vi "FGV Config.vi"(7 "Enum":enum16{"Read Config", "Save Config"}(ring)=enum."Save Config", 8 "error in":errorcluster, 10 "Config in":T1, 11 "config FName":string) -> (0 "error out":errorcluster, 2 "Config out":T1)   [LabVIEW 2012]
uses:
  controls/TP_Config.ctl
  <vilib>/Utility/config.llb/NI_LVConfig.lvlib
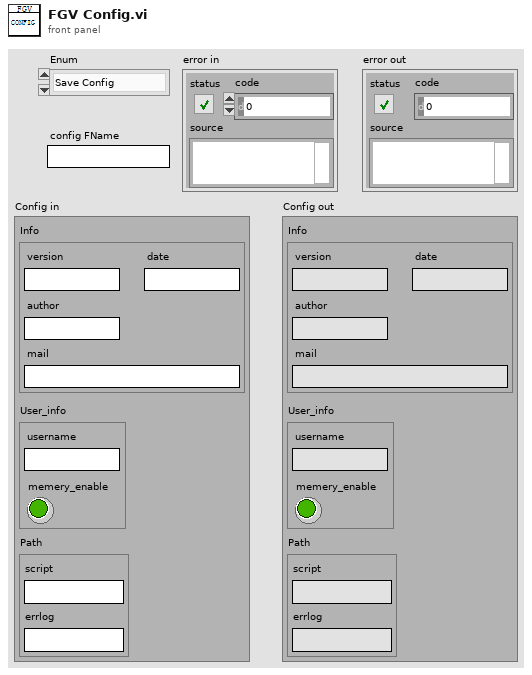
[diagram p1: front panel]
types:
  T1 = typedef "TP_Config.ctl" = cluster{"Info":cluster{"version":string, "date":string, "author":string, "mail":string}, "User_info":cluster{"username":string, "memery_enable":bool}, "Path":cluster{"script":string, "errlog":string}}
  T2 = typedef "NI_LVConfig.lvlib/Config Data RefNum.ctl" = refnum<k1>
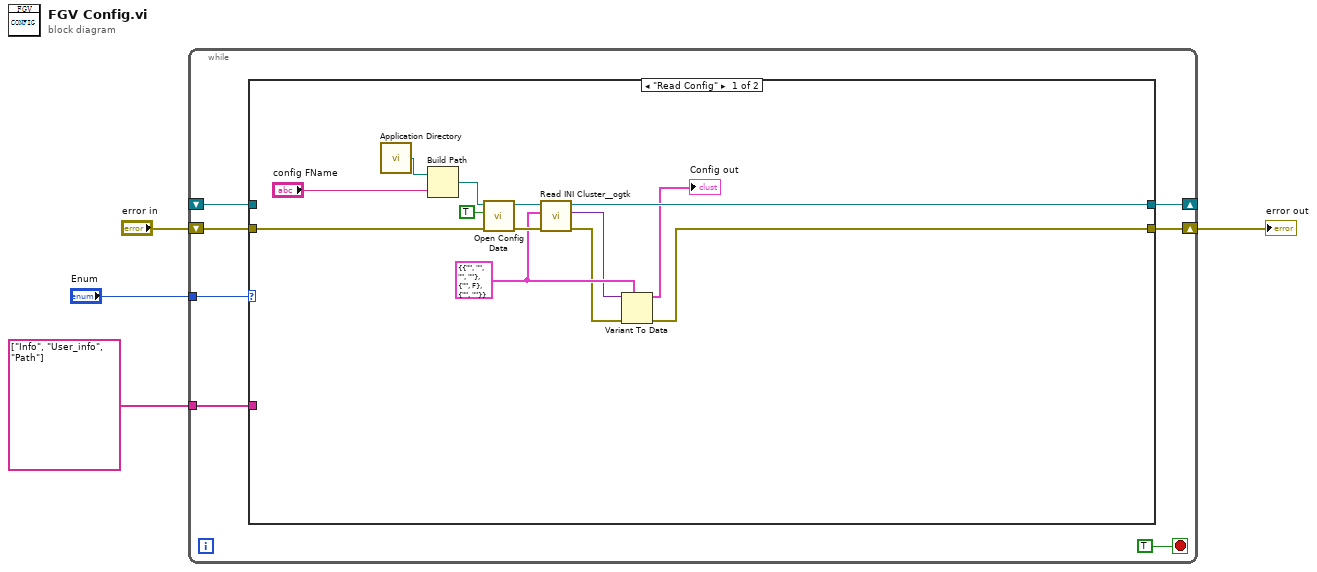
[diagram p0: block diagram]
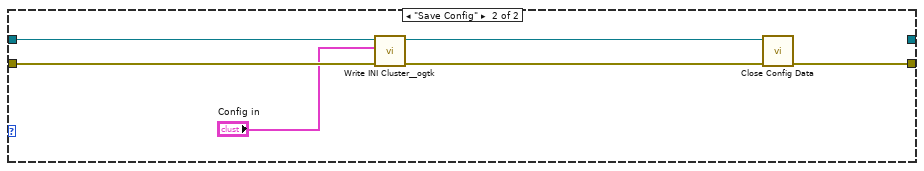
[diagram p2: hidden frame]
diagram:
  n1 = while {
    tunnel: "Enum" -> [w11]
    shift-right: [w9] -> _
    shift-left: _ -> [w10]
    shift-right: [w8] -> w2
    shift-left: "error in" -> [w7]
    tunnel: string[] ["Info", "User_info", "Path"] -> [w6]
    stop <- TRUE stop-if-true
    n2 = case shown="\"Read Config\"" w11 {
      tunnel: w10 -> [_ w26]
      tunnel: [w17 _] -> w9
      tunnel: [w12 w30] -> w8
      tunnel: w7 -> [w24 w27]
      tunnel: w6 -> [_ _]
      frame "Read Config" {
        w18 = T1 {"Info"={"version"="", "date"="", "author"="", "mail"=""}, "User_info"={"username"="", "memery_enable"=FALSE}, "Path"={"script"="", "errlog"=""}} ("Config")
        n3 = call <vilib>:"Application Directory.vi"() -> ("Application Directory"=w14:path)
        n4 = Build Path(base path=w14, name or relative path="config FName") -> (appended path=w22:path)
        n5 = call <vilib>:"Open Config Data.vi"("error in (no error)"=w24, "create file if necessary (T)"=TRUE, "configuration file path"=w22) -> ("error out"=w19:errorcluster, "refnum"=w20:T2)  [unwired: 6 in, 1 out]
        n6 = call <userlib>:"Read INI Cluster__ogtk.vi"("error in (no error)"=w19, "INI Fomatted Cluster Type"=w18, "refnum"=w20) -> ("error out"=w15:errorcluster, "INI Fomatted Cluster"=w16:variant, "dup refnum"=w17:T2)  [unwired: 4 in, 2 out]
        n7 = Variant To Data(error in=w15, type=w18, Variant=w16) -> (data=→"Config out":T1, error out=w12:errorcluster)
      }
      frame "Save Config" {
        n8 = call <userlib>:"Write INI Cluster__ogtk.vi"("error in (no error)"=w27, "INI Fomatted Cluster"="Config in", "refnum"=w26) -> ("error out"=w29:errorcluster, "dup refnum"=w28:T2)  [unwired: 7 in]
        n9 = call <vilib>:"Close Config Data.vi"("error in (no error)"=w29, "refnum"=w28) -> ("error out"=w30:errorcluster)  [unwired: 8 in, 1 out]
      }
    }
  }
  "error out" <- w2
